vi "2초 전진 90도 회전.vi"() -> ()   [LabVIEW 2015]
uses:
  <vilib>/NXT/LegoClasses/BrickReference/BrickReference.lvclass
  <vilib>/NXT/Subs/LVHSConnector.ctl
  <vilib>/NXT/NXTIO Xnodes/NXTIOXNode/NXTIO.xnode
  <vilib>/NXT/Dual Mode Library/Waits/Wait_Num.vi
  <vilib>/NXT/Dual Mode Library/Waits/Wait_Rotation.vi
  <vilib>/NXT/NXTIO Xnodes/NXTIONodeSubVIs/LEGOStopAllMotors.vi
  <vilib>/NXT/Block Support/NXT_OutputPort.ctl
  <vilib>/NXT/NXTIO Xnodes/NXTIONodeSubVIs/NXTMoveMotors.vi
panel:
  in  "Position Change (180) 2":i32=180
  in  "Port (Port A) 2":T1 items=["Port A", "Port B", "Port C", "Port D"]
  in  "Port (Port A)":T1 items=["Port A", "Port B", "Port C", "Port D"]
  in  "Position Change (180)":i32=180
  in  "Time (1 sec)":sgl=1.0
  in  "Power/Speed 2":i8=75
  out "NXT/EV3":T2
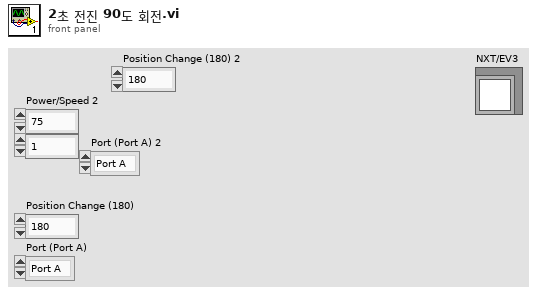
[diagram p1: front panel]
types:
  T1 = typedef "NXT_OutputPort.ctl" = u8
  T2 = typedef "LVHSConnector.ctl" = refnum<class "BrickReference.lvclass">
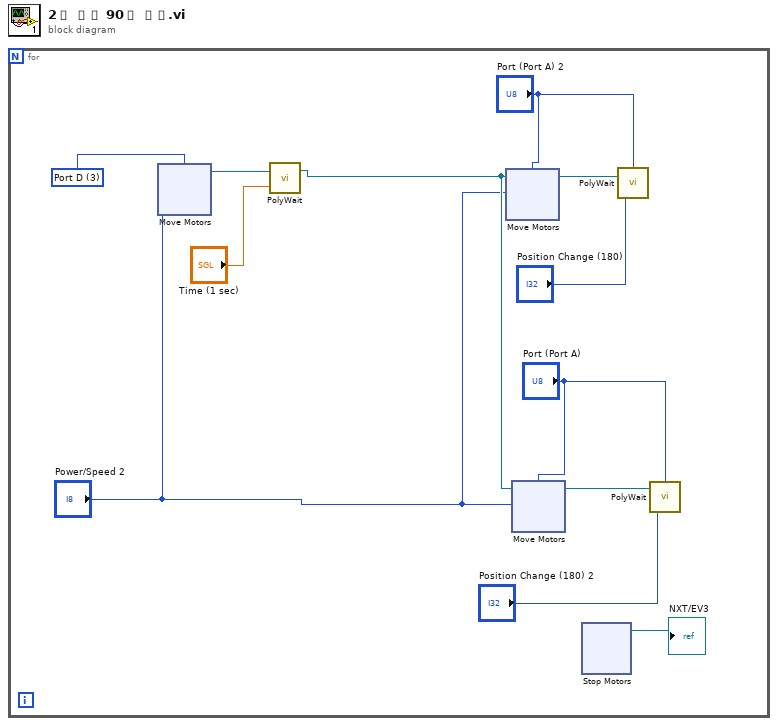
[diagram p0: block diagram]
diagram:
  n1 = for {
    w1 = T1 3 items=["Port A", "Port B", "Port C", "Port D"] ("Motors")
    n2 = xnode "Move Motors"("Power/Speed 1"="Power/Speed 2", "Motors"=w1) -> ("NXT/EV3"=w9:T2)  [unwired: 1 in]
    n3 = call-poly <vilib>:"PolyWait.vi"("Time (1 sec)"="Time (1 sec)", "NXT/EV3"=w9) -> ("NXT/EV3"=w6:T2)  [unwired: 2 in]
    n4 = xnode "Move Motors"("Power/Speed 1"="Power/Speed 2", "Motors"="Port (Port A) 2", "NXT/EV3"=w6) -> ("NXT/EV3"=w8:T2)
    n5 = xnode "Move Motors"("Power/Speed 1"="Power/Speed 2", "Motors"="Port (Port A)", "NXT/EV3"=w6) -> ("NXT/EV3"=w7:T2)
    n6 = xnode "Stop Motors"() -> ("NXT/EV3"=→"NXT/EV3":T2)  [unwired: 2 in]
    n7 = call-poly <vilib>:"PolyWait.vi"("Position Change (180)"="Position Change (180)", "NXT/EV3"=w8, "Port (Port A)"="Port (Port A) 2") -> ()  [unwired: 1 in, 1 out]
    n8 = call-poly <vilib>:"PolyWait.vi"("Position Change (180)"="Position Change (180) 2", "NXT/EV3"=w7, "Port (Port A)"="Port (Port A)") -> ()  [unwired: 1 in, 1 out]
  }
